vi "SendMessage.vi"(11 "Msg":string[](array[string])) -> ()   [LabVIEW 2018, in "TracerLibrary.lvlib" / "Tracer.lvclass"]
uses:
  Tracer.lvclass
  Tracer_ClassAttributes.vi
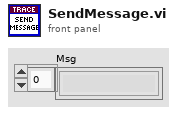
[diagram p1: front panel]
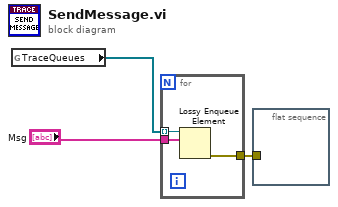
[diagram p0: block diagram]
diagram:
  n1 = global read "Tracer_ClassAttributes.vi" "TraceQueues"() -> (w1:refnum<queue>[])
  n2 = for {
    tunnel: w1 -> [w5] mode=indexing
    tunnel: [w6] -> w3
    tunnel: "Msg" -> [w4]
    n3 = Lossy Enqueue Element(queue=w5, element=w4) -> (error out=w6:errorcluster)  [unwired: 1 in, 3 out]
  }
  n4 = flat-sequence {
    tunnel: w3 -> [_]
    frame #0 {
    }
  }
